vi "核查数据发送(子VI).vi"(8 "错误输入":errorcluster) -> (0 "错误输出":errorcluster)   [LabVIEW 2016, in "数据传输系统-02.lvlib"]
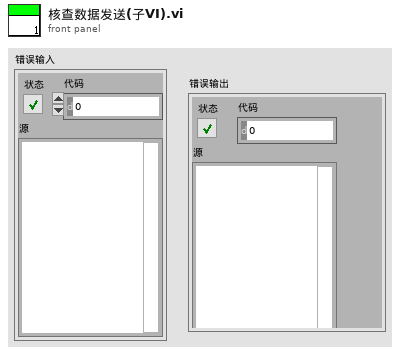
[diagram p1: front panel]
types:
  T1 = enum16{"质控数据", "操作日志", "仪器参数", "系统状态", "运行模式", "测量周期", "超标留样", "报警信息", "环境参数"}
  T2 = enum16{"空白测试", "跨度核查", "标样核查", "加标回收", "平行样", "集成干预"}
  T3 = cluster{"氨氮零点核查索引起始时间":string, "总磷零点核查索引起始时间":string, "总氮零点核查索引起始时间":string, "CODMn零点核查索引起始时间":string, "CODCr零点核查索引起始时间":string, "亚硝酸盐零点核查索引起始时间":string, "硫化物零点核查索引起始时间":string, "ORP零点核查索引起始时间":string}
  T4 = cluster{"[0]":string, "[1]":string, "[2]":string, "[3]":string, "[4]":string, "[5]":string, "[6]":string, "[7]":string}
  T5 = cluster{"PH":string[][], "CODCr":string[][], "氨氮":string[][], "CODMn":string[][], "总氮":string[][], "总磷":string[][], "电导率":string[][], "水温":string[][], "DO":string[][], "浊度":string[][], "叶绿素":string[][], "藻密度":string[][], "铜":string[][], "盐度":string[][], "水位":string[][], "流速":string[][], "瞬时流量":string[][], "累积流量":string[][], "亚硝酸盐":string[][], "硫化物":string[][], "ORP":string[][], "铅":string[][], "镉":string[][], "锌":string[][], "镍":string[][], "锰":string[][], "汞":string[][], "气温":string[][], "气压":string[][], "风速":string[][], "风向":string[][]}
  T6 = cluster{"氨氮跨度核查索引起始时间":string, "总磷跨度核查索引起始时间":string, "总氮跨度核查索引起始时间":string, "CODMn跨度核查索引起始时间":string, "CODCr跨度核查索引起始时间":string, "亚硝酸盐跨度核查索引起始时间":string, "硫化物跨度核查索引起始时间":string, "ORP跨度核查索引起始时间":string}
  T7 = cluster{"氨氮标样核查索引起始时间":string, "总磷标样核查索引起始时间":string, "总氮标样核查索引起始时间":string, "CODMn标样核查索引起始时间":string, "CODCr标样核查索引起始时间":string, "DO标样核查索引起始时间":string, "PH标样核查索引起始时间":string, "比电导率标样核查索引起始时间":string, "水温标样核查索引起始时间":string, "浊度标样核查索引起始时间":string, "叶绿素a标样核查索引起始时间":string, "藻密度标样核查索引起始时间":string, "亚硝酸盐标样核查索引起始时间":string, "硫化物标样核查索引起始时间":string, "ORP标样核查索引起始时间":string}
  T8 = cluster{"[0]":string, "[1]":string, "[2]":string, "[3]":string, "[4]":string, "[5]":string, "[6]":string, "[7]":string, "[8]":string, "[9]":string, "[10]":string, "[11]":string, "[12]":string, "[13]":string, "[14]":string}
  T9 = cluster{"氨氮加标回收索引起始时间":string, "总磷加标回收索引起始时间":string, "总氮加标回收索引起始时间":string, "CODMn加标回收索引起始时间":string, "CODCr加标回收索引起始时间":string}
  T10 = cluster{"[0]":string, "[1]":string, "[2]":string, "[3]":string, "[4]":string}
  T11 = cluster{"氨氮平行样索引起始时间":string, "总磷平行样索引起始时间":string, "总氮平行样索引起始时间":string, "CODMn平行样索引起始时间":string, "CODCr平行样索引起始时间":string}
  T12 = cluster{"氨氮集成干预索引起始时间":string, "总磷集成干预索引起始时间":string, "总氮集成干预索引起始时间":string, "CODMn集成干预索引起始时间":string, "CODCr集成干预索引起始时间":string, "DO集成干预索引起始时间":string, "PH集成干预索引起始时间":string, "比电导率集成干预索引起始时间":string, "水温集成干预索引起始时间":string, "浊度集成干预索引起始时间":string, "叶绿素a集成干预索引起始时间":string, "藻密度集成干预索引起始时间":string, "亚硝酸盐集成干预索引起始时间":string, "硫化物集成干预索引起始时间":string, "ORP集成干预索引起始时间":string}
  T13 = cluster{"氨氮仪器日志索引起始时间":string, "总磷仪器日志索引起始时间":string, "总氮仪器日志索引起始时间":string, "CODMn仪器日志索引起始时间":string, "CODCr仪器日志索引起始时间":string, "系统仪器日志索引起始时间":string}
  T14 = cluster{"[0]":string, "[1]":string, "[2]":string, "[3]":string, "[4]":string, "[5]":string}
  T15 = cluster{"氨氮仪器参数索引起始时间":string, "总磷仪器参数索引起始时间":string, "总氮仪器参数索引起始时间":string, "CODMn仪器参数索引起始时间":string, "CODCr仪器参数索引起始时间":string, "DO仪器参数索引起始时间":string, "PH仪器参数索引起始时间":string, "比电导率仪器参数索引起始时间":string, "水温仪器参数索引起始时间":string, "浊度仪器参数索引起始时间":string, "叶绿素a仪器参数索引起始时间":string, "藻密度仪器参数索引起始时间":string, "ORP仪器参数索引起始时间":string}
  T16 = cluster{"[0]":string, "[1]":string, "[2]":string, "[3]":string, "[4]":string, "[5]":string, "[6]":string, "[7]":string, "[8]":string, "[9]":string, "[10]":string, "[11]":string, "[12]":string}
  T17 = cluster{"氨氮报警信息索引起始时间":string, "总磷报警信息索引起始时间":string, "总氮报警信息索引起始时间":string, "CODMn报警信息索引起始时间":string, "CODCr报警信息索引起始时间":string, "DO报警信息索引起始时间":string, "PH报警信息索引起始时间":string, "比电导率报警信息索引起始时间":string, "水温报警信息索引起始时间":string, "浊度报警信息索引起始时间":string, "叶绿素报警信息索引起始时间":string, "系统报警信息索引起始时间":string}
  T18 = cluster{"[0]":string, "[1]":string, "[2]":string, "[3]":string, "[4]":string, "[5]":string, "[6]":string, "[7]":string, "[8]":string, "[9]":string, "[10]":string, "[11]":string}
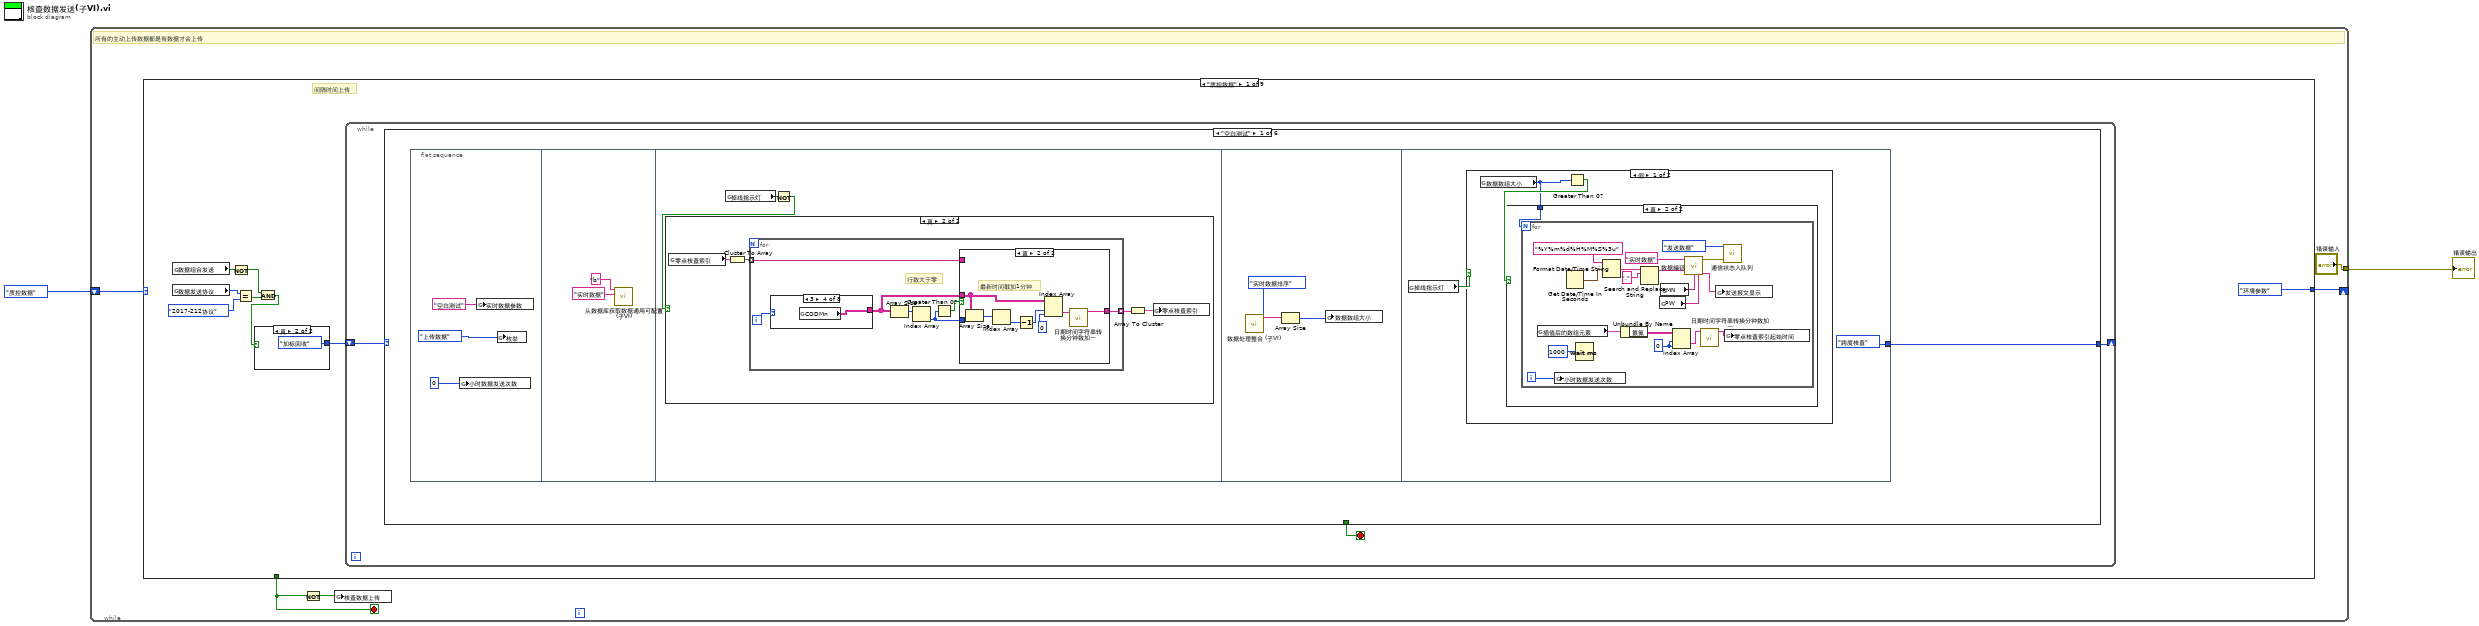
[diagram p0: block diagram]
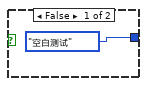
[diagram p2: hidden frame]
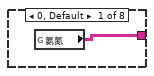
[diagram p4: hidden frame]
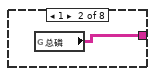
[diagram p5: hidden frame]
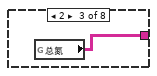
[diagram p6: hidden frame]
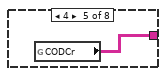
[diagram p7: hidden frame]
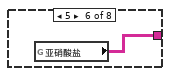
[diagram p8: hidden frame]
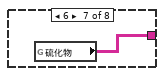
[diagram p9: hidden frame]
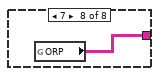
[diagram p10: hidden frame]
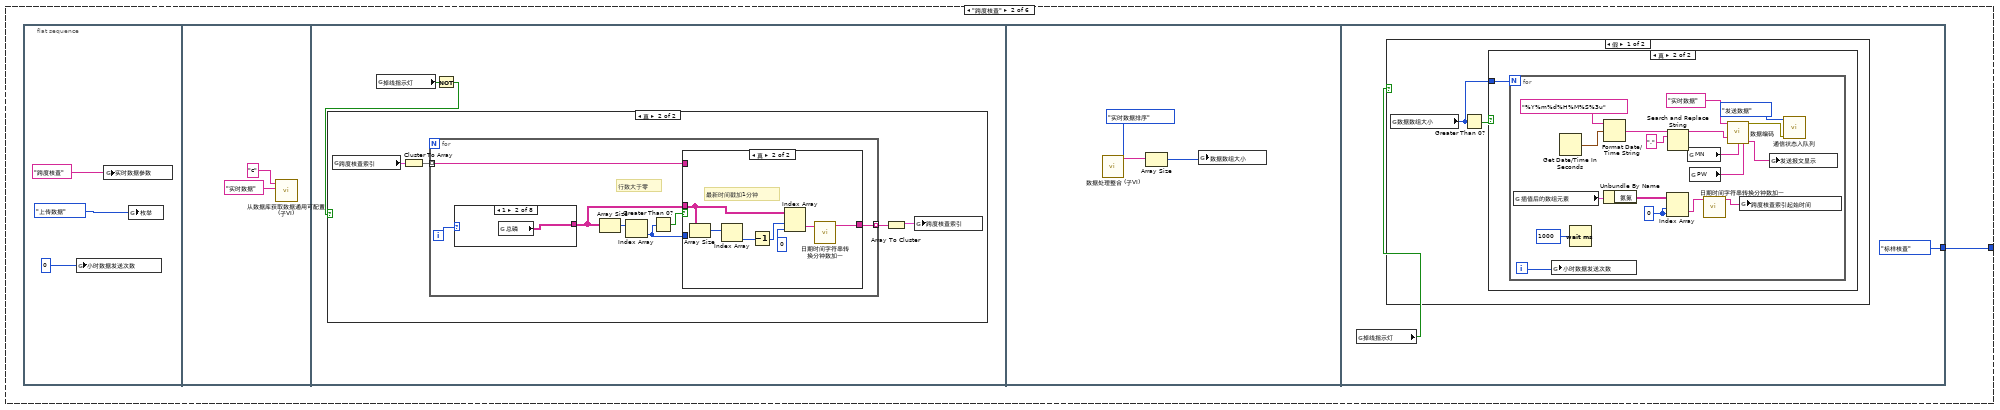
[diagram p14: hidden frame]
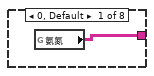
[diagram p16: hidden frame]
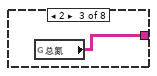
[diagram p17: hidden frame]
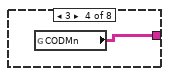
[diagram p18: hidden frame]
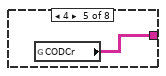
[diagram p19: hidden frame]
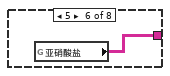
[diagram p20: hidden frame]
diagram:
  n1 = while "While循环" {
    shift-right: [w6] -> _
    shift-left: T1."质控数据" -> [w7]
    tunnel: ["错误输入"] -> w1
    stop <- w4 stop-if-true
    # "所有的主动上传数据都是有数据才会上传"
    n2 = case shown="\"质控数据\"" w7 {
      tunnel: [T1."环境参数" T1."仪器参数" T1."系统状态" T1."运行模式" T1."测量周期" T1."超标留样" T1."报警信息" T1."环境参数" T1."环境参数"] -> w6
      tunnel: [_ _ _ _ _ _ _ _ TRUE] -> w4
      frame "质控数据" {
        # "间隔时间上传"
        n3 = global read "断电保存全局.vi" "数据组合发送"() -> (w10:bool)
        n4 = global read "断电保存全局.vi" "数据发送协议"() -> (w13:enum16{"2005-212协议", "2017-212协议"})
        n5 = Not(x=w10) -> (.not. x?=w9:bool)
        n6 = Equal?(x=w13, y=enum16{"2005-212协议", "2017-212协议"}."2017-212协议" ("数据发送协议")) -> (x = y?=w11:bool)
        n7 = And(x=w9, y=w11) -> (x .and. y?=w8:bool)
        n8 = case shown="真" w8 {
          tunnel: [T2."空白测试" T2."加标回收"] -> w15
          frame False {
          }
          frame True {
          }
        }
        n9 = while {
          shift-right: [w18] -> _
          shift-left: w15 -> [w19]
          stop <- w20 stop-if-true
          n10 = case shown="\"空白测试\"" w19 {
            tunnel: [_ _ _ _ _ TRUE] -> w20
            tunnel: [w21 w82 w143 w211 w271 w324] -> w18
            frame "空白测试" {
              n11 = flat-sequence {
                tunnel: [T2."跨度核查"] -> w21
                frame #0 {
                  n12 = global write "全局 小时数据发送次数.vi" "小时数据发送次数"(0 ("小时数据发送次数")) -> ()
                  n13 = global write "全局 实时数据参数.vi" "实时数据参数"("空白测试") -> ()
                  n14 = global write "全局1.vi" "枚举"(enum16{"返回请求应答", "上传数据", "返回执行结果"}."上传数据" ("枚举")) -> ()
                }
                frame #1 {
                  n15 = call "从数据库获取数据通用可配置(子VI).vi"("table输入"="实时数据" ("新元素/子数组"), "列队名（唯一）"="b") -> ()  [unwired: 8 in, 2 out]
                }
                frame #2 {
                  n16 = global read "全局 数据发送重叠.vi" "掉线指示灯"() -> (w28:bool)
                  n17 = Not(x=w28) -> (.not. x?=w27:bool)
                  n18 = case shown="真" w27 {
                    frame False {
                    }
                    frame True {
                      n19 = global read "全局 时间2.vi" "零点核查索引"() -> (w32:T3)
                      n20 = Cluster To Array(cluster=w32) -> (array=w31:string[])
                      n21 = for {
                        tunnel: [w34] -> w30 mode=indexing
                        tunnel: w31 -> [w33] mode=indexing
                        i -> [w35]
                        # "行数大于零"
                        n22 = case shown="3" w35 {
                          tunnel: [w40 w41 w42 w43 w44 w45 w46 w47] -> w36
                          frame 0, Default {
                            n23 = global read "全局 所有参数.vi" "氨氮"() -> (w40:string[][])
                          }
                          frame 1 {
                            n24 = global read "全局 所有参数.vi" "总磷"() -> (w41:string[][])
                          }
                          frame 2 {
                            n25 = global read "全局 所有参数.vi" "总氮"() -> (w42:string[][])
                          }
                          frame 3 {
                            n26 = global read "全局 所有参数.vi" "CODMn"() -> (w43:string[][])
                          }
                          frame 4 {
                            n27 = global read "全局 所有参数.vi" "CODCr"() -> (w44:string[][])
                          }
                          frame 5 {
                            n28 = global read "全局 所有参数.vi" "亚硝酸盐"() -> (w45:string[][])
                          }
                          frame 6 {
                            n29 = global read "全局 所有参数.vi" "硫化物"() -> (w46:string[][])
                          }
                          frame 7 {
                            n30 = global read "全局 所有参数.vi" "ORP"() -> (w47:string[][])
                          }
                        }
                        n31 = Array Size(array=w36) -> (size(s)=w38:i32[])
                        n32 = Index Array(array=w38) -> (element=w37:i32)  [unwired: 1 in]
                        n33 = Greater Than 0?(x=w37) -> (x > 0?=w39:bool)
                        n34 = case shown="真" w39 {
                          tunnel: w37 -> [_ _]
                          tunnel: w36 -> [_ w51]
                          tunnel: [w48 w49] -> w34
                          tunnel: w33 -> [w48 _]
                          frame False {
                          }
                          frame True {
                            # "最新时间戳加1分钟"
                            n35 = Array Size(array=w51) -> (size(s)=w54:i32[])
                            n36 = Index Array(array=w54) -> (element=w53:i32)  [unwired: 1 in]
                            n37 = Decrement(x=w53) -> (x-1=w52:i32)
                            n38 = Index Array(array=w51, index (row)=w52, index (col)=0 ("禁用的索引 (列)")) -> (element=w55:string)
                            n39 = call "日期时间字符串转换分钟数加一.vi"("data[0]"=w55) -> ("日期/时间字符串"=w49:string)  [unwired: 10 in]
                          }
                        }
                      }
                      n40 = Array To Cluster(array=w30) -> (cluster=w29:T4)
                      n41 = global write "全局 时间2.vi" "零点核查索引"(w29) -> ()
                    }
                  }
                }
                frame #3 {
                  n42 = call "数据处理整合 (子VI).vi"("枚举"=enum16{"实时数据排序", "小时数据排序"}."实时数据排序") -> ("已排序的数组"=w58:string[])  [unwired: 10 in]
                  n43 = Array Size(array=w58) -> (size(s)=w57:i32)
                  n44 = global write "全局 数据数组大小.vi" "数据数组大小"(w57) -> ()
                }
                frame #4 {
                  n45 = global read "全局 数据发送重叠.vi" "掉线指示灯"() -> (w60:bool)
                  n46 = case shown="假" w60 {
                    frame False {
                      n47 = global read "全局 数据数组大小.vi" "数据数组大小"() -> (w61:i32)
                      n48 = Greater Than 0?(x=w61) -> (x > 0?=w62:bool)
                      n49 = case shown="真" w62 {
                        tunnel: w61 -> [_ w63]
                        frame False {
                        }
                        frame True {
                          n50 = for {
                            N: w63 -> [_]
                            i -> [w64]
                            w76 = 0 ("禁用的索引 (列)")
                            n51 = global read "插值后的新数组.vi" "插值后的数组元素"() -> (w80:T5)
                            n52 = global write "全局 小时数据发送次数.vi" "小时数据发送次数"(w64) -> ()
                            n53 = Get Date/Time In Seconds() -> (seconds since 1Jan1904=w68:timestamp)
                            n54 = Wait (ms)(milliseconds to wait=u32 1000 ("等待时间（毫秒）")) -> ()  [unwired: 1 out]
                            n55 = Format Date/Time String(time format string (%c)="%Y%m%d%H%M%S%3u" ("时间格式字符串(%c)"), seconds (now)=w68) -> (date/time string=w67:string)  [unwired: 1 in]
                            n56 = Unbundle By Name(w80) -> ("氨氮"=w79:string[][])
                            n57 = Search and Replace String(input string=w67, search string="." ("搜索字符串")) -> (result string=w65:string)  [unwired: 6 in, 3 out]
                            n58 = global read "断电保存全局.vi" "PW"() -> (w72:string)
                            n59 = global read "断电保存全局.vi" "MN"() -> (w73:string)
                            n60 = Index Array(array=w79, index (row)=w76, index (col)=w76) -> (element=w78:string)
                            n61 = call "数据编码.vi"("table输入"="实时数据" ("新元素/子数组"), "QN"=w65, "MN"=w73, "PW"=w72) -> ("错误常量"=w71:errorcluster, "通讯包字符串"=w75:string)  [unwired: 10 in]
                            n62 = call "日期时间字符串转换分钟数加一.vi"("data[0]"=w78) -> ("日期/时间字符串"=w77:string)  [unwired: 10 in]
                            n63 = global write "全局1.vi" "发送报文显示"(w75) -> ()
                            n64 = call "通信状态入队列.vi"("错误输入（无错误）"=w71, "枚举"=enum16{"打开连接", "发送数据", "读取数据", "数据处理", "关闭连接"}."发送数据") -> ()  [unwired: 9 in, 1 out]
                            n65 = global write "全局 时间2.vi" "零点核查索引起始时间"(w77) -> ()
                          }
                        }
                      }
                    }
                    frame True {
                    }
                  }
                }
              }
            }
            frame "跨度核查" {
              n66 = flat-sequence {
                tunnel: [T2."标样核查"] -> w82
                frame #0 {
                  n67 = global write "全局 小时数据发送次数.vi" "小时数据发送次数"(0 ("小时数据发送次数")) -> ()
                  n68 = global write "全局 实时数据参数.vi" "实时数据参数"("跨度核查") -> ()
                  n69 = global write "全局1.vi" "枚举"(enum16{"返回请求应答", "上传数据", "返回执行结果"}."上传数据" ("枚举")) -> ()
                }
                frame #1 {
                  n70 = call "从数据库获取数据通用可配置(子VI).vi"("table输入"="实时数据" ("新元素/子数组"), "列队名（唯一）"="c") -> ()  [unwired: 8 in, 2 out]
                }
                frame #2 {
                  n71 = global read "全局 数据发送重叠.vi" "掉线指示灯"() -> (w89:bool)
                  n72 = Not(x=w89) -> (.not. x?=w88:bool)
                  n73 = case shown="真" w88 {
                    frame False {
                    }
                    frame True {
                      n74 = global read "全局 时间2.vi" "跨度核查索引"() -> (w93:T6)
                      n75 = Cluster To Array(cluster=w93) -> (array=w92:string[])
                      n76 = for {
                        tunnel: [w95] -> w91 mode=indexing
                        tunnel: w92 -> [w94] mode=indexing
                        i -> [w96]
                        # "行数大于零"
                        n77 = case shown="1" w96 {
                          tunnel: [w101 w102 w103 w104 w105 w106 w107 w108] -> w97
                          frame 0, Default {
                            n78 = global read "全局 所有参数.vi" "氨氮"() -> (w101:string[][])
                          }
                          frame 1 {
                            n79 = global read "全局 所有参数.vi" "总磷"() -> (w102:string[][])
                          }
                          frame 2 {
                            n80 = global read "全局 所有参数.vi" "总氮"() -> (w103:string[][])
                          }
                          frame 3 {
                            n81 = global read "全局 所有参数.vi" "CODMn"() -> (w104:string[][])
                          }
                          frame 4 {
                            n82 = global read "全局 所有参数.vi" "CODCr"() -> (w105:string[][])
                          }
                          frame 5 {
                            n83 = global read "全局 所有参数.vi" "亚硝酸盐"() -> (w106:string[][])
                          }
                          frame 6 {
                            n84 = global read "全局 所有参数.vi" "硫化物"() -> (w107:string[][])
                          }
                          frame 7 {
                            n85 = global read "全局 所有参数.vi" "ORP"() -> (w108:string[][])
                          }
                        }
                        n86 = Array Size(array=w97) -> (size(s)=w99:i32[])
                        n87 = Index Array(array=w99) -> (element=w98:i32)  [unwired: 1 in]
                        n88 = Greater Than 0?(x=w98) -> (x > 0?=w100:bool)
                        n89 = case shown="真" w100 {
                          tunnel: w98 -> [_ _]
                          tunnel: w97 -> [_ w112]
                          tunnel: [w109 w110] -> w95
                          tunnel: w94 -> [w109 _]
                          frame False {
                          }
                          frame True {
                            # "最新时间戳加1分钟"
                            n90 = Array Size(array=w112) -> (size(s)=w115:i32[])
                            n91 = Index Array(array=w115) -> (element=w114:i32)  [unwired: 1 in]
                            n92 = Decrement(x=w114) -> (x-1=w113:i32)
                            n93 = Index Array(array=w112, index (row)=w113, index (col)=0 ("禁用的索引 (列)")) -> (element=w116:string)
                            n94 = call "日期时间字符串转换分钟数加一.vi"("data[0]"=w116) -> ("日期/时间字符串"=w110:string)  [unwired: 10 in]
                          }
                        }
                      }
                      n95 = Array To Cluster(array=w91) -> (cluster=w90:T4)
                      n96 = global write "全局 时间2.vi" "跨度核查索引"(w90) -> ()
                    }
                  }
                }
                frame #3 {
                  n97 = call "数据处理整合 (子VI).vi"("枚举"=enum16{"实时数据排序", "小时数据排序"}."实时数据排序") -> ("已排序的数组"=w119:string[])  [unwired: 10 in]
                  n98 = Array Size(array=w119) -> (size(s)=w118:i32)
                  n99 = global write "全局 数据数组大小.vi" "数据数组大小"(w118) -> ()
                }
                frame #4 {
                  n100 = global read "全局 数据发送重叠.vi" "掉线指示灯"() -> (w121:bool)
                  n101 = case shown="假" w121 {
                    frame False {
                      n102 = global read "全局 数据数组大小.vi" "数据数组大小"() -> (w122:i32)
                      n103 = Greater Than 0?(x=w122) -> (x > 0?=w123:bool)
                      n104 = case shown="真" w123 {
                        tunnel: w122 -> [_ w124]
                        frame False {
                        }
                        frame True {
                          n105 = for {
                            N: w124 -> [_]
                            i -> [w125]
                            w137 = 0 ("禁用的索引 (列)")
                            n106 = global read "插值后的新数组.vi" "插值后的数组元素"() -> (w141:T5)
                            n107 = global write "全局 小时数据发送次数.vi" "小时数据发送次数"(w125) -> ()
                            n108 = Get Date/Time In Seconds() -> (seconds since 1Jan1904=w129:timestamp)
                            n109 = Wait (ms)(milliseconds to wait=u32 1000 ("等待时间（毫秒）")) -> ()  [unwired: 1 out]
                            n110 = Format Date/Time String(time format string (%c)="%Y%m%d%H%M%S%3u" ("时间格式字符串(%c)"), seconds (now)=w129) -> (date/time string=w128:string)  [unwired: 1 in]
                            n111 = Unbundle By Name(w141) -> ("氨氮"=w140:string[][])
                            n112 = Index Array(array=w140, index (row)=w137, index (col)=w137) -> (element=w139:string)
                            n113 = Search and Replace String(input string=w128, search string="." ("搜索字符串")) -> (result string=w126:string)  [unwired: 6 in, 3 out]
                            n114 = global read "断电保存全局.vi" "MN"() -> (w135:string)
                            n115 = global read "断电保存全局.vi" "PW"() -> (w134:string)
                            n116 = call "日期时间字符串转换分钟数加一.vi"("data[0]"=w139) -> ("日期/时间字符串"=w138:string)  [unwired: 10 in]
                            n117 = call "数据编码.vi"("table输入"="实时数据" ("新元素/子数组"), "QN"=w126, "MN"=w135, "PW"=w134) -> ("错误常量"=w132:errorcluster, "通讯包字符串"=w133:string)  [unwired: 10 in]
                            n118 = global write "全局 时间2.vi" "跨度核查索引起始时间"(w138) -> ()
                            n119 = global write "全局1.vi" "发送报文显示"(w133) -> ()
                            n120 = call "通信状态入队列.vi"("错误输入（无错误）"=w132, "枚举"=enum16{"打开连接", "发送数据", "读取数据", "数据处理", "关闭连接"}."发送数据") -> ()  [unwired: 9 in, 1 out]
                          }
                        }
                      }
                    }
                    frame True {
                    }
                  }
                }
              }
            }
            frame "标样核查" {
              n121 = flat-sequence {
                tunnel: [T2."加标回收"] -> w143
                frame #0 {
                  n122 = global write "全局 小时数据发送次数.vi" "小时数据发送次数"(0 ("小时数据发送次数")) -> ()
                  n123 = global write "全局 实时数据参数.vi" "实时数据参数"("核查数据") -> ()
                  n124 = global write "全局1.vi" "枚举"(enum16{"返回请求应答", "上传数据", "返回执行结果"}."上传数据" ("枚举")) -> ()
                }
                frame #1 {
                  n125 = call "从数据库获取数据通用可配置(子VI).vi"("table输入"="实时数据" ("新元素/子数组"), "列队名（唯一）"="n") -> ()  [unwired: 8 in, 2 out]
                }
                frame #2 {
                  n126 = global read "全局 数据发送重叠.vi" "掉线指示灯"() -> (w150:bool)
                  n127 = Not(x=w150) -> (.not. x?=w149:bool)
                  n128 = case shown="真" w149 {
                    frame False {
                    }
                    frame True {
                      n129 = global read "全局 时间2.vi" "标样核查索引"() -> (w154:T7)
                      n130 = Cluster To Array(cluster=w154) -> (array=w153:string[])
                      n131 = for {
                        tunnel: [w156] -> w151 mode=indexing
                        tunnel: w153 -> [w155] mode=indexing
                        i -> [w157]
                        # "行数大于零"
                        n132 = case shown="0, 默认" w157 {
                          tunnel: [w162 w163 w164 w165 w166 w167 w168 w169 w170 w171 w172 w173 w174 w175 w176] -> w158
                          frame 0, Default {
                            n133 = global read "全局 所有参数.vi" "氨氮"() -> (w162:string[][])
                          }
                          frame 1 {
                            n134 = global read "全局 所有参数.vi" "总磷"() -> (w163:string[][])
                          }
                          frame 2 {
                            n135 = global read "全局 所有参数.vi" "总氮"() -> (w164:string[][])
                          }
                          frame 3 {
                            n136 = global read "全局 所有参数.vi" "CODMn"() -> (w165:string[][])
                          }
                          frame 4 {
                            n137 = global read "全局 所有参数.vi" "CODCr"() -> (w166:string[][])
                          }
                          frame 5 {
                            n138 = global read "全局 所有参数.vi" "DO"() -> (w167:string[][])
                          }
                          frame 6 {
                            n139 = global read "全局 所有参数.vi" "PH"() -> (w168:string[][])
                          }
                          frame 7 {
                            n140 = global read "全局 所有参数.vi" "电导率"() -> (w169:string[][])
                          }
                          frame 8 {
                            n141 = global read "全局 所有参数.vi" "水温"() -> (w170:string[][])
                          }
                          frame 9 {
                            n142 = global read "全局 所有参数.vi" "浊度"() -> (w171:string[][])
                          }
                          frame 10 {
                            n143 = global read "全局 所有参数.vi" "叶绿素"() -> (w172:string[][])
                          }
                          frame 11 {
                            n144 = global read "全局 所有参数.vi" "藻密度"() -> (w173:string[][])
                          }
                          frame 12 {
                            n145 = global read "全局 所有参数.vi" "亚硝酸盐"() -> (w174:string[][])
                          }
                          frame 13 {
                            n146 = global read "全局 所有参数.vi" "硫化物"() -> (w175:string[][])
                          }
                          frame 14 {
                            n147 = global read "全局 所有参数.vi" "ORP"() -> (w176:string[][])
                          }
                        }
                        n148 = Array Size(array=w158) -> (size(s)=w160:i32[])
                        n149 = Index Array(array=w160) -> (element=w159:i32)  [unwired: 1 in]
                        n150 = Greater Than 0?(x=w159) -> (x > 0?=w161:bool)
                        n151 = case shown="真" w161 {
                          tunnel: w157 -> [_ _]
                          tunnel: w159 -> [_ _]
                          tunnel: w158 -> [_ w179]
                          tunnel: [w177 w178] -> w156
                          tunnel: w155 -> [w177 _]
                          frame False {
                          }
                          frame True {
                            # "最新时间戳加1分钟"
                            n152 = Array Size(array=w179) -> (size(s)=w183:i32[])
                            n153 = Index Array(array=w183) -> (element=w182:i32)  [unwired: 1 in]
                            n154 = Decrement(x=w182) -> (x-1=w181:i32)
                            n155 = Index Array(array=w179, index (row)=w181, index (col)=0 ("禁用的索引 (列)")) -> (element=w184:string)
                            n156 = call "日期时间字符串转换分钟数加一.vi"("data[0]"=w184) -> ("日期/时间字符串"=w178:string)  [unwired: 10 in]
                          }
                        }
                      }
                      n157 = Array To Cluster(array=w151) -> (cluster=w152:T8)
                      n158 = global write "全局 时间2.vi" "标样核查索引"(w152) -> ()
                    }
                  }
                }
                frame #3 {
                  n159 = call "数据处理整合 (子VI).vi"("枚举"=enum16{"实时数据排序", "小时数据排序"}."实时数据排序") -> ("已排序的数组"=w187:string[])  [unwired: 10 in]
                  n160 = Array Size(array=w187) -> (size(s)=w186:i32)
                  n161 = global write "全局 数据数组大小.vi" "数据数组大小"(w186) -> ()
                }
                frame #4 {
                  n162 = global read "全局 数据发送重叠.vi" "掉线指示灯"() -> (w189:bool)
                  n163 = case shown="假" w189 {
                    frame False {
                      n164 = global read "全局 数据数组大小.vi" "数据数组大小"() -> (w190:i32)
                      n165 = Greater Than 0?(x=w190) -> (x > 0?=w191:bool)
                      n166 = case shown="真" w191 {
                        tunnel: w190 -> [_ w192]
                        frame False {
                        }
                        frame True {
                          n167 = for {
                            N: w192 -> [_]
                            i -> [w193]
                            w205 = 0 ("禁用的索引 (列)")
                            n168 = global read "插值后的新数组.vi" "插值后的数组元素"() -> (w209:T5)
                            n169 = Get Date/Time In Seconds() -> (seconds since 1Jan1904=w197:timestamp)
                            n170 = Wait (ms)(milliseconds to wait=u32 1000 ("等待时间（毫秒）")) -> ()  [unwired: 1 out]
                            n171 = Format Date/Time String(time format string (%c)="%Y%m%d%H%M%S%3u" ("时间格式字符串(%c)"), seconds (now)=w197) -> (date/time string=w196:string)  [unwired: 1 in]
                            n172 = Unbundle By Name(w209) -> ("氨氮"=w208:string[][])
                            n173 = global write "全局 小时数据发送次数.vi" "小时数据发送次数"(w193) -> ()
                            n174 = global read "断电保存全局.vi" "MN"() -> (w202:string)
                            n175 = Search and Replace String(input string=w196, search string="." ("搜索字符串")) -> (result string=w194:string)  [unwired: 6 in, 3 out]
                            n176 = global read "断电保存全局.vi" "PW"() -> (w201:string)
                            n177 = Index Array(array=w208, index (row)=w205, index (col)=w205) -> (element=w207:string)
                            n178 = call "日期时间字符串转换分钟数加一.vi"("data[0]"=w207) -> ("日期/时间字符串"=w206:string)  [unwired: 10 in]
                            n179 = call "数据编码.vi"("table输入"="实时数据" ("新元素/子数组"), "QN"=w194, "MN"=w202, "PW"=w201) -> ("错误常量"=w200:errorcluster, "通讯包字符串"=w204:string)  [unwired: 10 in]
                            n180 = global write "全局 时间2.vi" "标样核查索引起始时间"(w206) -> ()
                            n181 = global write "全局1.vi" "发送报文显示"(w204) -> ()
                            n182 = call "通信状态入队列.vi"("错误输入（无错误）"=w200, "枚举"=enum16{"打开连接", "发送数据", "读取数据", "数据处理", "关闭连接"}."发送数据") -> ()  [unwired: 9 in, 1 out]
                          }
                        }
                      }
                    }
                    frame True {
                    }
                  }
                }
              }
            }
            frame "加标回收" {
              n183 = flat-sequence {
                tunnel: [T2."平行样"] -> w211
                frame #0 {
                  n184 = global write "全局 小时数据发送次数.vi" "小时数据发送次数"(0 ("小时数据发送次数")) -> ()
                  n185 = global write "全局 实时数据参数.vi" "实时数据参数"("加标回收测试") -> ()
                  n186 = global write "全局1.vi" "枚举"(enum16{"返回请求应答", "上传数据", "返回执行结果"}."上传数据" ("枚举")) -> ()
                }
                frame #1 {
                  n187 = call "从数据库获取数据通用可配置(子VI).vi"("table输入"="加标回收" ("新元素/子数组"), "列队名（唯一）"="d") -> ()  [unwired: 8 in, 2 out]
                }
                frame #2 {
                  n188 = global read "全局 数据发送重叠.vi" "掉线指示灯"() -> (w218:bool)
                  n189 = Not(x=w218) -> (.not. x?=w217:bool)
                  n190 = case shown="真" w217 {
                    frame False {
                    }
                    frame True {
                      n191 = global read "全局 时间2.vi" "加标回收索引"() -> (w222:T9)
                      n192 = Cluster To Array(cluster=w222) -> (array=w221:string[])
                      n193 = for {
                        tunnel: [w224] -> w219 mode=indexing
                        tunnel: w221 -> [w223] mode=indexing
                        i -> [w225]
                        # "行数大于零"
                        n194 = case shown="0, 默认" w225 {
                          tunnel: [w230 w231 w232 w233 w234] -> w226
                          frame 0, Default {
                            n195 = global read "全局 所有参数.vi" "氨氮加标回收率"() -> (w230:string[][])
                          }
                          frame 1 {
                            n196 = global read "全局 所有参数.vi" "总磷加标回收率"() -> (w231:string[][])
                          }
                          frame 2 {
                            n197 = global read "全局 所有参数.vi" "总氮加标回收率"() -> (w232:string[][])
                          }
                          frame 3 {
                            n198 = global read "全局 所有参数.vi" "CODMn加标回收率"() -> (w233:string[][])
                          }
                          frame 4 {
                            n199 = global read "全局 所有参数.vi" "CODCr加标回收率"() -> (w234:string[][])
                          }
                        }
                        n200 = Array Size(array=w226) -> (size(s)=w228:i32[])
                        n201 = Index Array(array=w228) -> (element=w227:i32)  [unwired: 1 in]
                        n202 = Greater Than 0?(x=w227) -> (x > 0?=w229:bool)
                        n203 = case shown="真" w229 {
                          tunnel: w225 -> [_ _]
                          tunnel: w227 -> [_ _]
                          tunnel: w226 -> [_ w239]
                          tunnel: [w235 w236] -> w224
                          tunnel: w223 -> [w235 _]
                          frame False {
                          }
                          frame True {
                            # "最新时间戳加1分钟"
                            n204 = Array Size(array=w239) -> (size(s)=w241:i32[])
                            n205 = Index Array(array=w241) -> (element=w240:i32)  [unwired: 1 in]
                            n206 = Decrement(x=w240) -> (x-1=w238:i32)
                            n207 = Index Array(array=w239, index (row)=w238, index (col)=0 ("禁用的索引 (列)")) -> (element=w242:string)
                            n208 = call "日期时间字符串转换分钟数加一.vi"("data[0]"=w242) -> ("日期/时间字符串"=w236:string)  [unwired: 10 in]
                          }
                        }
                      }
                      n209 = Array To Cluster(array=w219) -> (cluster=w220:T10)
                      n210 = global write "全局 时间2.vi" "加标回收索引"(w220) -> ()
                    }
                  }
                }
                frame #3 {
                  n211 = call "加标回收数据处理整合 (子VI).vi"("枚举"=enum16{"实时数据排序", "小时数据排序"}."实时数据排序") -> ("已排序的数组"=w244:string[])  [unwired: 10 in]
                  n212 = Array Size(array=w244) -> (size(s)=w245:i32)
                  n213 = global write "全局 数据数组大小.vi" "数据数组大小"(w245) -> ()
                }
                frame #4 {
                  n214 = global read "全局 数据发送重叠.vi" "掉线指示灯"() -> (w247:bool)
                  n215 = case shown="假" w247 {
                    frame False {
                      n216 = global read "全局 数据数组大小.vi" "数据数组大小"() -> (w248:i32)
                      n217 = Greater Than 0?(x=w248) -> (x > 0?=w249:bool)
                      n218 = case shown="真" w249 {
                        tunnel: w248 -> [_ w250]
                        frame False {
                        }
                        frame True {
                          n219 = for {
                            N: w250 -> [_]
                            i -> [w251]
                            n220 = global read "全局 数据数组大小.vi" "数据数组大小"() -> (w266:i32)
                            n221 = global read "插值后的新数组.vi" "插值后的数组元素"() -> (w269:T5)
                            n222 = Get Date/Time In Seconds() -> (seconds since 1Jan1904=w255:timestamp)
                            n223 = Format Date/Time String(time format string (%c)="%Y%m%d%H%M%S%3u" ("时间格式字符串(%c)"), seconds (now)=w255) -> (date/time string=w254:string)  [unwired: 1 in]
                            n224 = Decrement(x=w266) -> (x-1=w265:i32)
                            n225 = Unbundle By Name(w269) -> ("氨氮"=w268:string[][])
                            n226 = Search and Replace String(input string=w254, search string="." ("搜索字符串")) -> (result string=w252:string)  [unwired: 6 in, 3 out]
                            n227 = global write "全局 小时数据发送次数.vi" "小时数据发送次数"(w251) -> ()
                            n228 = global read "断电保存全局.vi" "MN"() -> (w260:string)
                            n229 = Index Array(array=w268, index (row)=w265, index (col)=0 ("禁用的索引 (列)")) -> (element=w264:string)
                            n230 = global read "断电保存全局.vi" "PW"() -> (w259:string)
                            n231 = call "日期时间字符串转换分钟数加一.vi"("data[0]"=w264) -> ("日期/时间字符串"=w263:string)  [unwired: 10 in]
                            n232 = call "数据编码.vi"("table输入"="实时数据" ("新元素/子数组"), "QN"=w252, "MN"=w260, "PW"=w259) -> ("错误常量"=w258:errorcluster, "通讯包字符串"=w262:string)  [unwired: 10 in]
                            n233 = global write "全局 时间2.vi" "加标回收索引起始时间"(w263) -> ()
                            n234 = global write "全局1.vi" "发送报文显示"(w262) -> ()
                            n235 = call "通信状态入队列.vi"("错误输入（无错误）"=w258, "枚举"=enum16{"打开连接", "发送数据", "读取数据", "数据处理", "关闭连接"}."发送数据") -> ()  [unwired: 9 in, 1 out]
                            n236 = Wait (ms)(milliseconds to wait=u32 1000 ("等待时间（毫秒）")) -> ()  [unwired: 1 out]
                          }
                        }
                      }
                    }
                    frame True {
                    }
                  }
                }
              }
            }
            frame "平行样" {
              n237 = flat-sequence {
                tunnel: [T2."集成干预"] -> w271
                frame #0 {
                  n238 = global write "全局 小时数据发送次数.vi" "小时数据发送次数"(0 ("小时数据发送次数")) -> ()
                  n239 = global write "全局 实时数据参数.vi" "实时数据参数"("平行样测试") -> ()
                  n240 = global write "全局1.vi" "枚举"(enum16{"返回请求应答", "上传数据", "返回执行结果"}."上传数据" ("枚举")) -> ()
                }
                frame #1 {
                  n241 = call "从数据库获取数据通用可配置(子VI).vi"("table输入"="平行样测试" ("新元素/子数组"), "列队名（唯一）"="e") -> ()  [unwired: 8 in, 2 out]
                }
                frame #2 {
                  n242 = global read "全局 数据发送重叠.vi" "掉线指示灯"() -> (w278:bool)
                  n243 = Not(x=w278) -> (.not. x?=w277:bool)
                  n244 = case shown="真" w277 {
                    frame False {
                    }
                    frame True {
                      n245 = global read "全局 时间2.vi" "平行样索引"() -> (w282:T11)
                      n246 = Cluster To Array(cluster=w282) -> (array=w281:string[])
                      n247 = for {
                        tunnel: [w284] -> w279 mode=indexing
                        tunnel: w281 -> [w283] mode=indexing
                        i -> [w285]
                        # "行数大于零"
                        n248 = case shown="4" w285 {
                          tunnel: [w290 w291 w292 w293 w294] -> w286
                          frame 0, Default {
                            n249 = global read "全局 所有参数.vi" "氨氮"() -> (w290:string[][])
                          }
                          frame 1 {
                            n250 = global read "全局 所有参数.vi" "总磷"() -> (w291:string[][])
                          }
                          frame 2 {
                            n251 = global read "全局 所有参数.vi" "总氮"() -> (w292:string[][])
                          }
                          frame 3 {
                            n252 = global read "全局 所有参数.vi" "CODMn"() -> (w293:string[][])
                          }
                          frame 4 {
                            n253 = global read "全局 所有参数.vi" "CODCr"() -> (w294:string[][])
                          }
                        }
                        n254 = Array Size(array=w286) -> (size(s)=w288:i32[])
                        n255 = Index Array(array=w288) -> (element=w287:i32)  [unwired: 1 in]
                        n256 = Greater Than 0?(x=w287) -> (x > 0?=w289:bool)
                        n257 = case shown="真" w289 {
                          tunnel: w285 -> [_ _]
                          tunnel: w287 -> [_ _]
                          tunnel: w286 -> [_ w299]
                          tunnel: [w295 w296] -> w284
                          tunnel: w283 -> [w295 _]
                          frame False {
                          }
                          frame True {
                            # "最新时间戳加1分钟"
                            n258 = Array Size(array=w299) -> (size(s)=w301:i32[])
                            n259 = Index Array(array=w301) -> (element=w300:i32)  [unwired: 1 in]
                            n260 = Decrement(x=w300) -> (x-1=w298:i32)
                            n261 = Index Array(array=w299, index (row)=w298, index (col)=0 ("禁用的索引 (列)")) -> (element=w302:string)
                            n262 = call "日期时间字符串转换分钟数加一.vi"("data[0]"=w302) -> ("日期/时间字符串"=w296:string)  [unwired: 10 in]
                          }
                        }
                      }
                      n263 = Array To Cluster(array=w279) -> (cluster=w280:T10)
                      n264 = global write "全局 时间2.vi" "平行样索引"(w280) -> ()
                    }
                  }
                }
                frame #3 {
                  n265 = call "数据处理整合 (子VI).vi"("枚举"=enum16{"实时数据排序", "小时数据排序"}."实时数据排序") -> ("已排序的数组"=w305:string[])  [unwired: 10 in]
                  n266 = Array Size(array=w305) -> (size(s)=w304:i32)
                  n267 = global write "全局 数据数组大小.vi" "数据数组大小"(w304) -> ()
                }
                frame #4 {
                  n268 = global read "全局 数据发送重叠.vi" "掉线指示灯"() -> (w306:bool)
                  n269 = case shown="假" w306 {
                    frame False {
                      n270 = global read "全局 数据数组大小.vi" "数据数组大小"() -> (w308:i32)
                      n271 = Greater Than 0?(x=w308) -> (x > 0?=w309:bool)
                      n272 = case shown="真" w309 {
                        tunnel: w308 -> [_ w310]
                        frame False {
                        }
                        frame True {
                          n273 = for {
                            N: w310 -> [_]
                            i -> [w311]
                            n274 = global write "全局 小时数据发送次数.vi" "小时数据发送次数"(w311) -> ()
                            n275 = Get Date/Time In Seconds() -> (seconds since 1Jan1904=w315:timestamp)
                            n276 = Format Date/Time String(time format string (%c)="%Y%m%d%H%M%S%3u" ("时间格式字符串(%c)"), seconds (now)=w315) -> (date/time string=w314:string)  [unwired: 1 in]
                            n277 = Search and Replace String(input string=w314, search string="." ("搜索字符串")) -> (result string=w312:string)  [unwired: 6 in, 3 out]
                            n278 = global read "断电保存全局.vi" "MN"() -> (w320:string)
                            n279 = global read "断电保存全局.vi" "PW"() -> (w319:string)
                            n280 = call "数据编码.vi"("table输入"="实时数据" ("新元素/子数组"), "QN"=w312, "MN"=w320, "PW"=w319) -> ("错误常量"=w318:errorcluster, "通讯包字符串"=w322:string)  [unwired: 10 in]
                            n281 = global write "全局1.vi" "发送报文显示"(w322) -> ()
                            n282 = call "通信状态入队列.vi"("错误输入（无错误）"=w318, "枚举"=enum16{"打开连接", "发送数据", "读取数据", "数据处理", "关闭连接"}."发送数据") -> ()  [unwired: 9 in, 1 out]
                            n283 = Wait (ms)(milliseconds to wait=u32 1000 ("等待时间（毫秒）")) -> ()  [unwired: 1 out]
                          }
                        }
                      }
                    }
                    frame True {
                    }
                  }
                }
              }
            }
            frame "集成干预" {
              n284 = flat-sequence {
                tunnel: [T2."集成干预"] -> w324
                frame #0 {
                  n285 = global write "全局 小时数据发送次数.vi" "小时数据发送次数"(0 ("小时数据发送次数")) -> ()
                  n286 = global write "全局 实时数据参数.vi" "实时数据参数"("集成干预测试") -> ()
                  n287 = global write "全局1.vi" "枚举"(enum16{"返回请求应答", "上传数据", "返回执行结果"}."上传数据" ("枚举")) -> ()
                }
                frame #1 {
                  n288 = call "从数据库获取数据通用可配置(子VI).vi"("table输入"="集成干预测试" ("新元素/子数组"), "列队名（唯一）"="f") -> ()  [unwired: 8 in, 2 out]
                }
                frame #2 {
                  n289 = global read "全局 数据发送重叠.vi" "掉线指示灯"() -> (w332:bool)
                  n290 = Not(x=w332) -> (.not. x?=w331:bool)
                  n291 = case shown="真" w331 {
                    frame False {
                    }
                    frame True {
                      n292 = global read "全局 时间2.vi" "集成干预索引"() -> (w336:T12)
                      n293 = Cluster To Array(cluster=w336) -> (array=w335:string[])
                      n294 = for {
                        tunnel: [w338] -> w333 mode=indexing
                        tunnel: w335 -> [w337] mode=indexing
                        i -> [w339]
                        # "行数大于零"
                        n295 = case shown="0, 默认" w339 {
                          tunnel: [w344 w345 w346 w347 w348 w349 w350 w351 w352 w353 w354 w355 w356 w357 w358] -> w340
                          frame 0, Default {
                            n296 = global read "全局 所有参数.vi" "氨氮"() -> (w344:string[][])
                          }
                          frame 1 {
                            n297 = global read "全局 所有参数.vi" "总磷"() -> (w345:string[][])
                          }
                          frame 2 {
                            n298 = global read "全局 所有参数.vi" "总氮"() -> (w346:string[][])
                          }
                          frame 3 {
                            n299 = global read "全局 所有参数.vi" "CODMn"() -> (w347:string[][])
                          }
                          frame 4 {
                            n300 = global read "全局 所有参数.vi" "CODCr"() -> (w348:string[][])
                          }
                          frame 5 {
                            n301 = global read "全局 所有参数.vi" "DO"() -> (w349:string[][])
                          }
                          frame 6 {
                            n302 = global read "全局 所有参数.vi" "PH"() -> (w350:string[][])
                          }
                          frame 7 {
                            n303 = global read "全局 所有参数.vi" "电导率"() -> (w351:string[][])
                          }
                          frame 8 {
                            n304 = global read "全局 所有参数.vi" "水温"() -> (w352:string[][])
                          }
                          frame 9 {
                            n305 = global read "全局 所有参数.vi" "浊度"() -> (w353:string[][])
                          }
                          frame 10 {
                            n306 = global read "全局 所有参数.vi" "叶绿素"() -> (w354:string[][])
                          }
                          frame 11 {
                            n307 = global read "全局 所有参数.vi" "藻密度"() -> (w355:string[][])
                          }
                          frame 12 {
                            n308 = global read "全局 所有参数.vi" "亚硝酸盐"() -> (w356:string[][])
                          }
                          frame 13 {
                            n309 = global read "全局 所有参数.vi" "硫化物"() -> (w357:string[][])
                          }
                          frame 14 {
                            n310 = global read "全局 所有参数.vi" "ORP"() -> (w358:string[][])
                          }
                        }
                        n311 = Array Size(array=w340) -> (size(s)=w342:i32[])
                        n312 = Index Array(array=w342) -> (element=w341:i32)  [unwired: 1 in]
                        n313 = Greater Than 0?(x=w341) -> (x > 0?=w343:bool)
                        n314 = case shown="真" w343 {
                          tunnel: w339 -> [_ _]
                          tunnel: w341 -> [_ _]
                          tunnel: w340 -> [_ w361]
                          tunnel: [w359 w360] -> w338
                          tunnel: w337 -> [w359 _]
                          frame False {
                          }
                          frame True {
                            # "最新时间戳加1分钟"
                            n315 = Array Size(array=w361) -> (size(s)=w365:i32[])
                            n316 = Index Array(array=w365) -> (element=w364:i32)  [unwired: 1 in]
                            n317 = Decrement(x=w364) -> (x-1=w363:i32)
                            n318 = Index Array(array=w361, index (row)=w363, index (col)=0 ("禁用的索引 (列)")) -> (element=w366:string)
                            n319 = call "日期时间字符串转换分钟数加一.vi"("data[0]"=w366) -> ("日期/时间字符串"=w360:string)  [unwired: 10 in]
                          }
                        }
                      }
                      n320 = Array To Cluster(array=w333) -> (cluster=w334:T8)
                      n321 = global write "全局 时间2.vi" "集成干预索引"(w334) -> ()
                    }
                  }
                }
                frame #3 {
                  n322 = call "数据处理整合 (子VI).vi"("枚举"=enum16{"实时数据排序", "小时数据排序"}."实时数据排序") -> ("已排序的数组"=w369:string[])  [unwired: 10 in]
                  n323 = Array Size(array=w369) -> (size(s)=w368:i32)
                  n324 = global write "全局 数据数组大小.vi" "数据数组大小"(w368) -> ()
                }
                frame #4 {
                  n325 = global read "全局 数据发送重叠.vi" "掉线指示灯"() -> (w371:bool)
                  n326 = case shown="假" w371 {
                    frame False {
                      n327 = global read "全局 数据数组大小.vi" "数据数组大小"() -> (w372:i32)
                      n328 = Greater Than 0?(x=w372) -> (x > 0?=w373:bool)
                      n329 = case shown="真" w373 {
                        tunnel: w372 -> [_ w374]
                        frame False {
                        }
                        frame True {
                          n330 = for {
                            N: w374 -> [_]
                            i -> [w375]
                            n331 = Get Date/Time In Seconds() -> (seconds since 1Jan1904=w379:timestamp)
                            n332 = Format Date/Time String(time format string (%c)="%Y%m%d%H%M%S%3u" ("时间格式字符串(%c)"), seconds (now)=w379) -> (date/time string=w378:string)  [unwired: 1 in]
                            n333 = global write "全局 小时数据发送次数.vi" "小时数据发送次数"(w375) -> ()
                            n334 = global read "断电保存全局.vi" "MN"() -> (w383:string)
                            n335 = global read "断电保存全局.vi" "PW"() -> (w382:string)
                            n336 = Search and Replace String(input string=w378, search string="." ("搜索字符串")) -> (result string=w376:string)  [unwired: 6 in, 3 out]
                            n337 = call "数据编码.vi"("table输入"="实时数据" ("新元素/子数组"), "QN"=w376, "MN"=w383, "PW"=w382) -> ("错误常量"=w384:errorcluster, "通讯包字符串"=w386:string)  [unwired: 10 in]
                            n338 = global write "全局1.vi" "发送报文显示"(w386) -> ()
                            n339 = call "通信状态入队列.vi"("错误输入（无错误）"=w384, "枚举"=enum16{"打开连接", "发送数据", "读取数据", "数据处理", "关闭连接"}."发送数据") -> ()  [unwired: 9 in, 1 out]
                            n340 = Wait (ms)(milliseconds to wait=u32 1000 ("等待时间（毫秒）")) -> ()  [unwired: 1 out]
                          }
                        }
                      }
                    }
                    frame True {
                    }
                  }
                }
              }
            }
          }
        }
      }
      frame "操作日志" {
        # "间隔时间上传"
        # "直接1分钟查询 一次,有数据就按数据上传,没数据就不上传,在数据发送那边有做处理"
        n341 = flat-sequence {
          frame #0 {
            # "时间"
            n342 = global write "全局 小时数据发送次数.vi" "小时数据发送次数"(0 ("小时数据发送次数")) -> ()
            n343 = call "日志信息主动发送(子VI).vi"() -> ()  [unwired: 12 in]
            n344 = global write "全局1.vi" "枚举"(enum16{"返回请求应答", "上传数据", "返回执行结果"}."上传数据" ("枚举")) -> ()
          }
          frame #1 {
            n345 = call "获取操作日志 (子VI).vi"("table输入"="操作日志") -> ()  [unwired: 11 in]
          }
          frame #2 {
            n346 = global read "全局 数据发送重叠.vi" "掉线指示灯"() -> (w393:bool)
            n347 = Not(x=w393) -> (.not. x?=w392:bool)
            n348 = case shown="真" w392 {
              frame False {
              }
              frame True {
                n349 = global read "全局 时间2.vi" "仪器日志索引"() -> (w397:T13)
                n350 = Cluster To Array(cluster=w397) -> (array=w396:string[])
                n351 = for {
                  tunnel: w396 -> [w398] mode=indexing
                  tunnel: [w399] -> w394 mode=indexing
                  i -> [w401]
                  # "行数大于零"
                  n352 = case shown="5" w401 {
                    tunnel: [w405 w406 w407 w408 w409 w410] -> w400
                    frame 0, Default {
                      n353 = global read "全局 所有参数.vi" "氨氮"() -> (w405:string[][])
                    }
                    frame 1 {
                      n354 = global read "全局 所有参数.vi" "总磷"() -> (w406:string[][])
                    }
                    frame 2 {
                      n355 = global read "全局 所有参数.vi" "总氮"() -> (w407:string[][])
                    }
                    frame 3 {
                      n356 = global read "全局 所有参数.vi" "CODMn"() -> (w408:string[][])
                    }
                    frame 4 {
                      n357 = global read "全局 所有参数.vi" "CODCr"() -> (w409:string[][])
                    }
                    frame 5 {
                      n358 = global read "全局 所有参数.vi" "DO"() -> (w410:string[][])
                    }
                  }
                  n359 = Array Size(array=w400) -> (size(s)=w403:i32[])
                  n360 = Index Array(array=w403) -> (element=w402:i32)  [unwired: 1 in]
                  n361 = Greater Than 0?(x=w402) -> (x > 0?=w404:bool)
                  n362 = case shown="真" w404 {
                    tunnel: w402 -> [_ _]
                    tunnel: w400 -> [_ w416]
                    tunnel: [w411 w412] -> w399
                    tunnel: w398 -> [w411 _]
                    frame False {
                    }
                    frame True {
                      # "最新时间戳加1分钟"
                      n363 = Array Size(array=w416) -> (size(s)=w418:i32[])
                      n364 = Index Array(array=w418) -> (element=w417:i32)  [unwired: 1 in]
                      n365 = Decrement(x=w417) -> (x-1=w415:i32)
                      n366 = Index Array(array=w416, index (row)=w415, index (col)=0 ("禁用的索引 (列)")) -> (element=w413:string)
                      n367 = call "日期时间字符串转换秒数加一.vi"("data[0]"=w413) -> ("日期/时间字符串"=w412:string)  [unwired: 10 in]
                    }
                  }
                }
                n368 = Array To Cluster(array=w394) -> (cluster=w395:T14)
                n369 = global write "全局 时间2.vi" "仪器日志索引"(w395) -> ()
              }
            }
          }
          frame #3 {
            n370 = call "数据处理整合 (子VI).vi"("枚举"=enum16{"实时数据排序", "小时数据排序"}."实时数据排序") -> ("已排序的数组"=w421:string[])  [unwired: 10 in]
            n371 = Array Size(array=w421) -> (size(s)=w420:i32)
            n372 = global write "全局 数据数组大小.vi" "数据数组大小"(w420) -> ()
          }
          frame #4 {
            # "判定是否存表"
            n373 = global read "全局 数据发送重叠.vi" "掉线指示灯"() -> (w422:bool)
            n374 = case shown="假" w422 {
              frame False {
                n375 = global read "全局 数据数组大小.vi" "数据数组大小"() -> (w423:i32)
                n376 = Greater Than 0?(x=w423) -> (x > 0?=w424:bool)
                n377 = case shown="真" w424 {
                  frame False {
                  }
                  frame True {
                    n378 = while {
                      stop <- w426 stop-if-true
                      n379 = Get Date/Time In Seconds() -> (seconds since 1Jan1904=w438:timestamp)
                      n380 = Format Date/Time String(time format string (%c)="%Y%m%d%H%M%S%3u" ("时间格式字符串(%c)"), seconds (now)=w438) -> (date/time string=w437:string)  [unwired: 1 in]
                      n381 = Search and Replace String(input string=w437, search string="." ("搜索字符串")) -> (result string=w435:string)  [unwired: 6 in, 3 out]
                      n382 = global read "断电保存全局.vi" "MN"() -> (w432:string)
                      n383 = global read "断电保存全局.vi" "PW"() -> (w431:string)
                      n384 = call "数据编码.vi"("table输入"="操作日志" ("新元素/子数组"), "QN"=w435, "MN"=w432, "PW"=w431) -> ("错误常量"=w430:errorcluster, "通讯包字符串"=w434:string)  [unwired: 10 in]
                      n385 = global read "全局 小时数据发送次数.vi" "小时数据发送次数"() -> (w427:i32)
                      n386 = global read "全局 数据数组大小.vi" "数据数组大小"() -> (w428:i32)
                      n387 = call "通信状态入队列.vi"("错误输入（无错误）"=w430, "枚举"=enum16{"打开连接", "发送数据", "读取数据", "数据处理", "关闭连接"}."发送数据") -> ()  [unwired: 9 in, 1 out]
                      n388 = global write "全局1.vi" "发送报文显示"(w434) -> ()
                      n389 = Decrement(x=w428) -> (x-1=w429:i32)
                      n390 = Greater Or Equal?(x=w427, y=w429) -> (x >= y?=w426:bool)
                      n391 = Wait (ms)(milliseconds to wait=u32 1000 ("等待时间（毫秒）")) -> ()  [unwired: 1 out]
                    }
                  }
                }
              }
              frame True {
              }
            }
          }
        }
      }
      frame "仪器参数" {
        # "间隔时间上传"
        # "直接1分钟查询 一次,有数据就按数据上传,没数据就不上传,在数据发送那边有做处理"
        n392 = flat-sequence {
          frame #0 {
            n393 = global write "全局 小时数据发送次数.vi" "小时数据发送次数"(0 ("小时数据发送次数")) -> ()
            n394 = global write "全局1.vi" "枚举"(enum16{"返回请求应答", "上传数据", "返回执行结果"}."上传数据" ("枚举")) -> ()
          }
          frame #1 {
            n395 = call "获取操作日志 (子VI).vi"("table输入"="仪器参数") -> ()  [unwired: 11 in]
          }
          frame #2 {
            n396 = global read "全局 数据发送重叠.vi" "掉线指示灯"() -> (w446:bool)
            n397 = Not(x=w446) -> (.not. x?=w445:bool)
            n398 = case shown="真" w445 {
              frame False {
              }
              frame True {
                n399 = global read "全局 时间2.vi" "仪器参数索引"() -> (w450:T15)
                n400 = Cluster To Array(cluster=w450) -> (array=w449:string[])
                n401 = for {
                  tunnel: [w454] -> w447 mode=indexing
                  tunnel: w449 -> [w453] mode=indexing
                  i -> [w452]
                  # "行数大于零"
                  n402 = case shown="12" w452 {
                    tunnel: [w458 w459 w460 w461 w462 w463 w464 w465 w466 w467 w468 w469 w470] -> w451
                    frame 0, Default {
                      n403 = global read "全局 所有参数.vi" "氨氮"() -> (w458:string[][])
                    }
                    frame 1 {
                      n404 = global read "全局 所有参数.vi" "总磷"() -> (w459:string[][])
                    }
                    frame 2 {
                      n405 = global read "全局 所有参数.vi" "总氮"() -> (w460:string[][])
                    }
                    frame 3 {
                      n406 = global read "全局 所有参数.vi" "CODMn"() -> (w461:string[][])
                    }
                    frame 4 {
                      n407 = global read "全局 所有参数.vi" "CODCr"() -> (w462:string[][])
                    }
                    frame 5 {
                      n408 = global read "全局 所有参数.vi" "DO"() -> (w463:string[][])
                    }
                    frame 6 {
                      n409 = global read "全局 所有参数.vi" "PH"() -> (w464:string[][])
                    }
                    frame 7 {
                      n410 = global read "全局 所有参数.vi" "电导率"() -> (w465:string[][])
                    }
                    frame 8 {
                      n411 = global read "全局 所有参数.vi" "水温"() -> (w466:string[][])
                    }
                    frame 9 {
                      n412 = global read "全局 所有参数.vi" "浊度"() -> (w467:string[][])
                    }
                    frame 10 {
                      n413 = global read "全局 所有参数.vi" "叶绿素"() -> (w468:string[][])
                    }
                    frame 11 {
                      n414 = global read "全局 所有参数.vi" "藻密度"() -> (w469:string[][])
                    }
                    frame 12 {
                      n415 = global read "全局 所有参数.vi" "ORP"() -> (w470:string[][])
                    }
                  }
                  n416 = Array Size(array=w451) -> (size(s)=w456:i32[])
                  n417 = Index Array(array=w456) -> (element=w455:i32)  [unwired: 1 in]
                  n418 = Greater Than 0?(x=w455) -> (x > 0?=w457:bool)
                  n419 = case shown="真" w457 {
                    tunnel: w455 -> [_ _]
                    tunnel: w451 -> [_ w475]
                    tunnel: [w471 w472] -> w454
                    tunnel: w453 -> [w471 _]
                    frame False {
                    }
                    frame True {
                      # "最新时间戳加1分钟"
                      n420 = Array Size(array=w475) -> (size(s)=w477:i32[])
                      n421 = Index Array(array=w477) -> (element=w476:i32)  [unwired: 1 in]
                      n422 = Decrement(x=w476) -> (x-1=w474:i32)
                      n423 = Index Array(array=w475, index (row)=w474, index (col)=0 ("禁用的索引 (列)")) -> (element=w478:string)
                      n424 = call "日期时间字符串转换分钟数加一.vi"("data[0]"=w478) -> ("日期/时间字符串"=w472:string)  [unwired: 10 in]
                    }
                  }
                }
                n425 = Array To Cluster(array=w447) -> (cluster=w448:T16)
                n426 = global write "全局 时间2.vi" "仪器参数索引"(w448) -> ()
              }
            }
          }
          frame #3 {
            n427 = call "数据处理整合 (子VI).vi"("枚举"=enum16{"实时数据排序", "小时数据排序"}."实时数据排序") -> ("已排序的数组"=w481:string[])  [unwired: 10 in]
            n428 = Array Size(array=w481) -> (size(s)=w480:i32)
            n429 = global write "全局 数据数组大小.vi" "数据数组大小"(w480) -> ()
          }
          frame #4 {
            # "判定是否存表"
            n430 = global read "全局 数据发送重叠.vi" "掉线指示灯"() -> (w482:bool)
            n431 = case shown="假" w482 {
              frame False {
                n432 = global read "全局 数据数组大小.vi" "数据数组大小"() -> (w483:i32)
                n433 = Greater Than 0?(x=w483) -> (x > 0?=w484:bool)
                n434 = case shown="真" w484 {
                  frame False {
                  }
                  frame True {
                    n435 = while {
                      stop <- w485 stop-if-true
                      n436 = Get Date/Time In Seconds() -> (seconds since 1Jan1904=w498:timestamp)
                      n437 = Format Date/Time String(time format string (%c)="%Y%m%d%H%M%S%3u" ("时间格式字符串(%c)"), seconds (now)=w498) -> (date/time string=w497:string)  [unwired: 1 in]
                      n438 = Search and Replace String(input string=w497, search string="." ("搜索字符串")) -> (result string=w495:string)  [unwired: 6 in, 3 out]
                      n439 = global read "断电保存全局.vi" "MN"() -> (w492:string)
                      n440 = global read "断电保存全局.vi" "PW"() -> (w491:string)
                      n441 = global read "全局 数据数组大小.vi" "数据数组大小"() -> (w487:i32)
                      n442 = call "数据编码.vi"("table输入"="仪器参数" ("新元素/子数组"), "QN"=w495, "MN"=w492, "PW"=w491) -> ("错误常量"=w490:errorcluster, "通讯包字符串"=w494:string)  [unwired: 10 in]
                      n443 = global read "全局 小时数据发送次数.vi" "小时数据发送次数"() -> (w488:i32)
                      n444 = global write "全局1.vi" "发送报文显示"(w494) -> ()
                      n445 = call "通信状态入队列.vi"("错误输入（无错误）"=w490, "枚举"=enum16{"打开连接", "发送数据", "读取数据", "数据处理", "关闭连接"}."发送数据") -> ()  [unwired: 9 in, 1 out]
                      n446 = Decrement(x=w487) -> (x-1=w486:i32)
                      n447 = Greater Or Equal?(x=w488, y=w486) -> (x >= y?=w485:bool)
                      n448 = Wait (ms)(milliseconds to wait=u32 1000 ("等待时间（毫秒）")) -> ()  [unwired: 1 out]
                    }
                  }
                }
              }
              frame True {
              }
            }
          }
        }
      }
      frame "系统状态" {
        # "直接1分钟查询 一次,有变化就按上传,没变化就不上传"
        n449 = flat-sequence {
          frame #0 {
            # "时间"
            n450 = global write "全局 小时数据发送次数.vi" "小时数据发送次数"(0 ("小时数据发送次数")) -> ()
            n451 = global write "全局 数据数组大小.vi" "数据数组大小"(1 ("数据数组大小")) -> ()
            n452 = global write "全局1.vi" "枚举"(enum16{"返回请求应答", "上传数据", "返回执行结果"}."上传数据" ("枚举")) -> ()
          }
          frame #1 {
            # "判定是否存表"
            n453 = global read "全局 数据发送重叠.vi" "掉线指示灯"() -> (w505:bool)
            n454 = case shown="假" w505 {
              frame False {
                n455 = global read "全局1.vi" "系统状态"() -> (w506:bool)
                n456 = case shown="真" w506 {
                  frame False {
                  }
                  frame True {
                    n457 = global read "全局 小时数据发送次数.vi" "小时数据发送次数"() -> (w514:i32)
                    n458 = global write "全局1.vi" "系统状态"(FALSE ("系统状态")) -> ()
                    n459 = Get Date/Time In Seconds() -> (seconds since 1Jan1904=w518:timestamp)
                    n460 = Increment(x=w514) -> (x+1=w513:i32)
                    n461 = Format Date/Time String(time format string (%c)="%Y%m%d%H%M%S%3u" ("时间格式字符串(%c)"), seconds (now)=w518) -> (date/time string=w517:string)  [unwired: 1 in]
                    n462 = global write "全局 小时数据发送次数.vi" "小时数据发送次数"(w513) -> ()
                    n463 = Search and Replace String(input string=w517, search string="." ("搜索字符串")) -> (result string=w515:string)  [unwired: 6 in, 3 out]
                    n464 = global read "断电保存全局.vi" "MN"() -> (w510:string)
                    n465 = global read "断电保存全局.vi" "PW"() -> (w509:string)
                    n466 = call "数据编码.vi"("table输入"="系统状态" ("新元素/子数组"), "QN"=w515, "MN"=w510, "PW"=w509) -> ("错误常量"=w508:errorcluster, "通讯包字符串"=w512:string)  [unwired: 10 in]
                    n467 = call "通信状态入队列.vi"("错误输入（无错误）"=w508, "枚举"=enum16{"打开连接", "发送数据", "读取数据", "数据处理", "关闭连接"}."发送数据") -> ()  [unwired: 9 in, 1 out]
                    n468 = global write "全局1.vi" "发送报文显示"(w512) -> ()
                  }
                }
              }
              frame True {
              }
            }
          }
        }
      }
      frame "运行模式" {
        # "直接1分钟查询 一次,有变化就按上传,没变化就不上传"
        n469 = flat-sequence {
          frame #0 {
            # "时间"
            n470 = global write "全局 小时数据发送次数.vi" "小时数据发送次数"(0 ("小时数据发送次数")) -> ()
            n471 = global write "全局 数据数组大小.vi" "数据数组大小"(1 ("数据数组大小")) -> ()
            n472 = global write "全局1.vi" "枚举"(enum16{"返回请求应答", "上传数据", "返回执行结果"}."上传数据" ("枚举")) -> ()
          }
          frame #1 {
            # "判定是否存表"
            n473 = global read "全局 数据发送重叠.vi" "掉线指示灯"() -> (w525:bool)
            n474 = case shown="假" w525 {
              frame False {
                n475 = global read "全局1.vi" "运行模式"() -> (w526:bool)
                n476 = case shown="真" w526 {
                  frame False {
                  }
                  frame True {
                    n477 = global read "全局 小时数据发送次数.vi" "小时数据发送次数"() -> (w534:i32)
                    n478 = global write "全局1.vi" "运行模式"(FALSE ("系统状态")) -> ()
                    n479 = Get Date/Time In Seconds() -> (seconds since 1Jan1904=w538:timestamp)
                    n480 = Increment(x=w534) -> (x+1=w533:i32)
                    n481 = Format Date/Time String(time format string (%c)="%Y%m%d%H%M%S%3u" ("时间格式字符串(%c)"), seconds (now)=w538) -> (date/time string=w537:string)  [unwired: 1 in]
                    n482 = global write "全局 小时数据发送次数.vi" "小时数据发送次数"(w533) -> ()
                    n483 = Search and Replace String(input string=w537, search string="." ("搜索字符串")) -> (result string=w535:string)  [unwired: 6 in, 3 out]
                    n484 = global read "断电保存全局.vi" "MN"() -> (w530:string)
                    n485 = global read "断电保存全局.vi" "PW"() -> (w529:string)
                    n486 = call "数据编码.vi"("table输入"="运行模式" ("新元素/子数组"), "QN"=w535, "MN"=w530, "PW"=w529) -> ("错误常量"=w528:errorcluster, "通讯包字符串"=w532:string)  [unwired: 10 in]
                    n487 = call "通信状态入队列.vi"("错误输入（无错误）"=w528, "枚举"=enum16{"打开连接", "发送数据", "读取数据", "数据处理", "关闭连接"}."发送数据") -> ()  [unwired: 9 in, 1 out]
                    n488 = global write "全局1.vi" "发送报文显示"(w532) -> ()
                  }
                }
              }
              frame True {
              }
            }
          }
        }
      }
      frame "测量周期" {
        # "直接1分钟查询 一次,有变化就按上传,没变化就不上传"
        n489 = flat-sequence {
          frame #0 {
            # "时间"
            n490 = global write "全局 小时数据发送次数.vi" "小时数据发送次数"(0 ("小时数据发送次数")) -> ()
            n491 = global write "全局 数据数组大小.vi" "数据数组大小"(1 ("数据数组大小")) -> ()
            n492 = global write "全局1.vi" "枚举"(enum16{"返回请求应答", "上传数据", "返回执行结果"}."上传数据" ("枚举")) -> ()
          }
          frame #1 {
            # "判定是否存表"
            n493 = global read "全局 数据发送重叠.vi" "掉线指示灯"() -> (w545:bool)
            n494 = case shown="假" w545 {
              frame False {
                n495 = global read "全局1.vi" "测量周期"() -> (w546:bool)
                n496 = case shown="真" w546 {
                  frame False {
                  }
                  frame True {
                    n497 = global read "全局 小时数据发送次数.vi" "小时数据发送次数"() -> (w554:i32)
                    n498 = global write "全局1.vi" "测量周期"(FALSE ("系统状态")) -> ()
                    n499 = Get Date/Time In Seconds() -> (seconds since 1Jan1904=w558:timestamp)
                    n500 = Increment(x=w554) -> (x+1=w553:i32)
                    n501 = Format Date/Time String(time format string (%c)="%Y%m%d%H%M%S%3u" ("时间格式字符串(%c)"), seconds (now)=w558) -> (date/time string=w557:string)  [unwired: 1 in]
                    n502 = global write "全局 小时数据发送次数.vi" "小时数据发送次数"(w553) -> ()
                    n503 = Search and Replace String(input string=w557, search string="." ("搜索字符串")) -> (result string=w555:string)  [unwired: 6 in, 3 out]
                    n504 = global read "断电保存全局.vi" "MN"() -> (w550:string)
                    n505 = global read "断电保存全局.vi" "PW"() -> (w549:string)
                    n506 = call "数据编码.vi"("table输入"="测量周期" ("新元素/子数组"), "QN"=w555, "MN"=w550, "PW"=w549) -> ("错误常量"=w548:errorcluster, "通讯包字符串"=w552:string)  [unwired: 10 in]
                    n507 = global write "全局1.vi" "发送报文显示"(w552) -> ()
                    n508 = call "通信状态入队列.vi"("错误输入（无错误）"=w548, "枚举"=enum16{"打开连接", "发送数据", "读取数据", "数据处理", "关闭连接"}."发送数据") -> ()  [unwired: 9 in, 1 out]
                  }
                }
              }
              frame True {
              }
            }
          }
        }
      }
      frame "超标留样" {
        # "直接1分钟查询 一次,有变化就按上传,没变化就不上传"
        n509 = flat-sequence {
          frame #0 {
            # "时间"
            n510 = global write "全局 小时数据发送次数.vi" "小时数据发送次数"(0 ("小时数据发送次数")) -> ()
            n511 = global write "全局 数据数组大小.vi" "数据数组大小"(1 ("数据数组大小")) -> ()
            n512 = global write "全局1.vi" "枚举"(enum16{"返回请求应答", "上传数据", "返回执行结果"}."上传数据" ("枚举")) -> ()
          }
          frame #1 {
            # "判定是否存表"
            n513 = global read "全局 数据发送重叠.vi" "掉线指示灯"() -> (w565:bool)
            n514 = case shown="假" w565 {
              frame False {
                n515 = global read "全局1.vi" "超标留样"() -> (w566:bool)
                n516 = case shown="真" w566 {
                  frame False {
                  }
                  frame True {
                    n517 = global read "全局 小时数据发送次数.vi" "小时数据发送次数"() -> (w574:i32)
                    n518 = global write "全局1.vi" "超标留样"(FALSE ("系统状态")) -> ()
                    n519 = Get Date/Time In Seconds() -> (seconds since 1Jan1904=w578:timestamp)
                    n520 = Increment(x=w574) -> (x+1=w573:i32)
                    n521 = Format Date/Time String(time format string (%c)="%Y%m%d%H%M%S%3u" ("时间格式字符串(%c)"), seconds (now)=w578) -> (date/time string=w577:string)  [unwired: 1 in]
                    n522 = global write "全局 小时数据发送次数.vi" "小时数据发送次数"(w573) -> ()
                    n523 = Search and Replace String(input string=w577, search string="." ("搜索字符串")) -> (result string=w575:string)  [unwired: 6 in, 3 out]
                    n524 = global read "断电保存全局.vi" "MN"() -> (w569:string)
                    n525 = global read "断电保存全局.vi" "PW"() -> (w568:string)
                    n526 = call "数据编码.vi"("table输入"="超标留样" ("新元素/子数组"), "QN"=w575, "MN"=w569, "PW"=w568) -> ("错误常量"=w570:errorcluster, "通讯包字符串"=w572:string)  [unwired: 10 in]
                    n527 = global write "全局1.vi" "发送报文显示"(w572) -> ()
                    n528 = call "通信状态入队列.vi"("错误输入（无错误）"=w570, "枚举"=enum16{"打开连接", "发送数据", "读取数据", "数据处理", "关闭连接"}."发送数据") -> ()  [unwired: 9 in, 1 out]
                  }
                }
              }
              frame True {
              }
            }
          }
        }
      }
      frame "报警信息" {
        # "间隔时间上传"
        # "直接1分钟查询 一次,有数据就按数据上传,没数据为空的不传,在数据发送那边有做处理"
        n529 = flat-sequence {
          frame #0 {
            # "分钟时间间隔"
            n530 = call "日志信息主动发送(子VI).vi"() -> ()  [unwired: 12 in]
            n531 = global write "全局 小时数据发送次数.vi" "小时数据发送次数"(0 ("小时数据发送次数")) -> ()
            n532 = global write "全局1.vi" "枚举"(enum16{"返回请求应答", "上传数据", "返回执行结果"}."上传数据" ("枚举")) -> ()
          }
          frame #1 {
            n533 = call "获取报警信息 (子VI).vi"() -> ()  [unwired: 12 in]
          }
          frame #2 {
            n534 = global read "全局 数据发送重叠.vi" "掉线指示灯"() -> (w585:bool)
            n535 = Not(x=w585) -> (.not. x?=w584:bool)
            n536 = case shown="真" w584 {
              frame False {
              }
              frame True {
                n537 = global read "全局 时间2.vi" "报警信息索引"() -> (w589:T17)
                n538 = Cluster To Array(cluster=w589) -> (array=w588:string[])
                n539 = for {
                  tunnel: [w591] -> w586 mode=indexing
                  tunnel: w588 -> [w590] mode=indexing
                  i -> [w593]
                  # "行数大于零"
                  n540 = case shown="1" w593 {
                    tunnel: [w597 w598 w599 w600 w601 w602 w603 w604 w605 w606 w607 w608] -> w592
                    frame 0, Default {
                      n541 = global read "全局 所有参数.vi" "氨氮"() -> (w597:string[][])
                    }
                    frame 1 {
                      n542 = global read "全局 所有参数.vi" "总磷"() -> (w598:string[][])
                    }
                    frame 2 {
                      n543 = global read "全局 所有参数.vi" "总氮"() -> (w599:string[][])
                    }
                    frame 3 {
                      n544 = global read "全局 所有参数.vi" "CODMn"() -> (w600:string[][])
                    }
                    frame 4 {
                      n545 = global read "全局 所有参数.vi" "CODCr"() -> (w601:string[][])
                    }
                    frame 5 {
                      n546 = global read "全局 所有参数.vi" "DO"() -> (w602:string[][])
                    }
                    frame 6 {
                      n547 = global read "全局 所有参数.vi" "PH"() -> (w603:string[][])
                    }
                    frame 7 {
                      n548 = global read "全局 所有参数.vi" "电导率"() -> (w604:string[][])
                    }
                    frame 8 {
                      n549 = global read "全局 所有参数.vi" "水温"() -> (w605:string[][])
                    }
                    frame 9 {
                      n550 = global read "全局 所有参数.vi" "浊度"() -> (w606:string[][])
                    }
                    frame 10 {
                      n551 = global read "全局 所有参数.vi" "叶绿素"() -> (w607:string[][])
                    }
                    frame 11 {
                      n552 = global read "全局 所有参数.vi" "藻密度"() -> (w608:string[][])
                    }
                  }
                  n553 = Array Size(array=w592) -> (size(s)=w595:i32[])
                  n554 = Index Array(array=w595) -> (element=w594:i32)  [unwired: 1 in]
                  n555 = Greater Than 0?(x=w594) -> (x > 0?=w596:bool)
                  n556 = case shown="真" w596 {
                    tunnel: w594 -> [_ _]
                    tunnel: w592 -> [_ w613]
                    tunnel: [w609 w610] -> w591
                    tunnel: w590 -> [w609 _]
                    frame False {
                    }
                    frame True {
                      # "最新时间戳加1分钟"
                      n557 = Array Size(array=w613) -> (size(s)=w615:i32[])
                      n558 = Index Array(array=w615) -> (element=w614:i32)  [unwired: 1 in]
                      n559 = Decrement(x=w614) -> (x-1=w612:i32)
                      n560 = Index Array(array=w613, index (row)=w612, index (col)=0 ("禁用的索引 (列)")) -> (element=w616:string)
                      n561 = call "日期时间字符串转换分钟数加一.vi"("data[0]"=w616) -> ("日期/时间字符串"=w610:string)  [unwired: 10 in]
                    }
                  }
                }
                n562 = Array To Cluster(array=w586) -> (cluster=w587:T18)
                n563 = global write "全局 时间2.vi" "报警信息索引"(w587) -> ()
              }
            }
          }
          frame #3 {
            n564 = call "数据处理整合 (子VI).vi"("枚举"=enum16{"实时数据排序", "小时数据排序"}."实时数据排序") -> ("已排序的数组"=w619:string[])  [unwired: 10 in]
            n565 = Array Size(array=w619) -> (size(s)=w618:i32)
            n566 = global write "全局 数据数组大小.vi" "数据数组大小"(w618) -> ()
          }
          frame #4 {
            # "判定是否存表"
            n567 = global read "全局 数据发送重叠.vi" "掉线指示灯"() -> (w620:bool)
            n568 = case shown="假" w620 {
              frame False {
                # "判定数据不为空才发"
                n569 = global read "全局 数据数组大小.vi" "数据数组大小"() -> (w621:i32)
                n570 = Greater Than 0?(x=w621) -> (x > 0?=w622:bool)
                n571 = case shown="真" w622 {
                  frame False {
                    n572 = global write "全局1.vi" "核查数据上传"(FALSE ("数据上传")) -> ()
                  }
                  frame True {
                    n573 = while {
                      stop <- w625 stop-if-true
                      n574 = Wait (ms)(milliseconds to wait=u32 1000 ("等待时间（毫秒）")) -> ()  [unwired: 1 out]
                      n575 = Get Date/Time In Seconds() -> (seconds since 1Jan1904=w637:timestamp)
                      n576 = Format Date/Time String(time format string (%c)="%Y%m%d%H%M%S%3u" ("时间格式字符串(%c)"), seconds (now)=w637) -> (date/time string=w636:string)  [unwired: 1 in]
                      n577 = global read "全局 数据数组大小.vi" "数据数组大小"() -> (w627:i32)
                      n578 = Search and Replace String(input string=w636, search string="." ("搜索字符串")) -> (result string=w634:string)  [unwired: 6 in, 3 out]
                      n579 = global read "断电保存全局.vi" "MN"() -> (w631:string)
                      n580 = global read "断电保存全局.vi" "PW"() -> (w630:string)
                      n581 = global read "全局 小时数据发送次数.vi" "小时数据发送次数"() -> (w628:i32)
                      n582 = call "数据编码.vi"("table输入"="报警信息" ("新元素/子数组"), "QN"=w634, "MN"=w631, "PW"=w630) -> ("错误常量"=w629:errorcluster, "通讯包字符串"=w633:string)  [unwired: 10 in]
                      n583 = Decrement(x=w627) -> (x-1=w626:i32)
                      n584 = global write "全局1.vi" "发送报文显示"(w633) -> ()
                      n585 = Greater Or Equal?(x=w628, y=w626) -> (x >= y?=w625:bool)
                      n586 = call "通信状态入队列.vi"("错误输入（无错误）"=w629, "枚举"=enum16{"打开连接", "发送数据", "读取数据", "数据处理", "关闭连接"}."发送数据") -> ()  [unwired: 9 in, 1 out]
                    }
                  }
                }
              }
              frame True {
              }
            }
          }
        }
      }
      frame "环境参数" {
        n587 = call "核查数据断电保存 (子VI).vi"() -> ()  [unwired: 12 in]
      }
    }
    n588 = Not(x=w4) -> (.not. x?=w5:bool)
    n589 = global write "全局1.vi" "核查数据上传"(w5) -> ()
  }
  "错误输出" <- w1
